vi "Set Inline Buffer.vi"(8 "error in (no error)":errorcluster, 10 "Command Parameters":T1, 11 "Dispatcher in":refnum<class "Dispatcher Thread.lvclass">) -> (0 "error out":errorcluster, 3 "Dispatcher out":refnum<class "Dispatcher Thread.lvclass">)   [LabVIEW 2019, in "DSF Core.lvlib" / "Dispatcher Thread.lvclass"]
uses:
  Dispatcher Thread.lvclass
  Interface/Dispatcher/Parameters.ctl
  Dispatcher Thread.lvclass/Dispatcher Thread.ctl
  Interface/Dispatcher/Inline Buffer Parameters.ctl
  Interface/Plugin/Plugin Interface.lvclass
  Interface/Dispatcher/Dispatcher Interface.lvclass
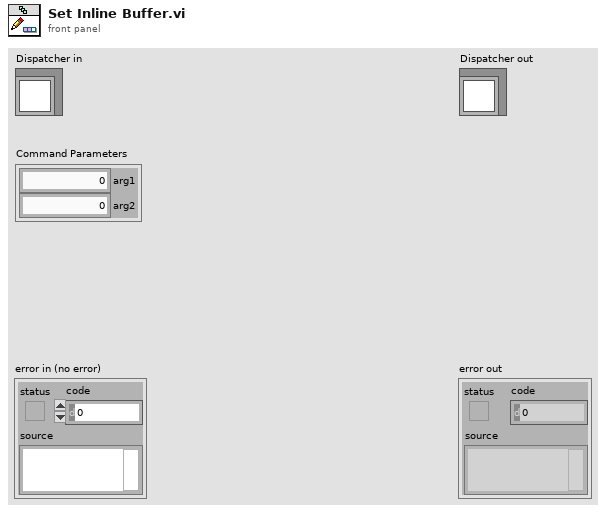
[diagram p1: front panel]
types:
  T1 = typedef "DSF Core.lvlib/Dispatcher Interface.lvclass/Parameters.ctl" = cluster{"arg1":u64, "arg2":u64}
  T2 = typedef "DSF Core.lvlib/Dispatcher Interface.lvclass/Inline Buffer Parameters.ctl" = cluster{"address":u64, "size":u64}
  T3 = typedef "DSF Core.lvlib/Dispatcher Thread.lvclass/Plugin Settings.ctl" = cluster{"Transfer Group threads":i32[], "Plugin Thread Interfaces":refnum<class "Plugin Interface.lvclass">[]}
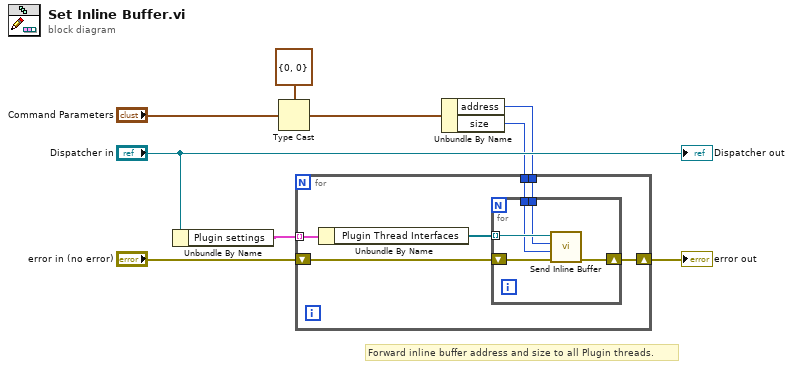
[diagram p0: block diagram]
diagram:
  # "Forward inline buffer address and size to all Plugin threads."
  n1 = Unbundle By Name("Dispatcher in") -> ("Plugin settings"=w9:T3[])
  n2 = Type Cast(type=T2 {"address"=0, "size"=0} ("Inline Buffer Parameters"), x="Command Parameters") -> (*(type *) &x=w2:T2)
  n3 = Unbundle By Name(w2) -> ("address"=w5:u64, "size"=w4:u64)
  n4 = for {
    tunnel: w9 -> [w11] mode=indexing
    shift-right: [w15] -> w6
    shift-left: "error in (no error)" -> [w14]
    tunnel: w4 -> [w13]
    tunnel: w5 -> [w12]
    n5 = Unbundle By Name(w11) -> ("Plugin Thread Interfaces"=w10:refnum<class "Plugin Interface.lvclass">[])
    n6 = for {
      tunnel: w10 -> [w20] mode=indexing
      shift-right: [w19] -> w15
      shift-left: w14 -> [w18]
      tunnel: w13 -> [w16]
      tunnel: w12 -> [w17]
      n7 = call "Send Inline Buffer.vi"("error in (no error)"=w18, "size"=w16, "address"=w17, "Plugin Interface in"=w20) -> ("error out"=w19:errorcluster)  [unwired: 6 in, 1 out]
    }
  }
  "error out" <- w6
  "Dispatcher out" <- "Dispatcher in"
